vi "2283_catapulta.vi"(1 "swithLimit":bool, 2 "Reset":bool, 3 "catapulta":bool) -> (0 "motor":i32)   [LabVIEW 2015]
uses:
  TypeDefs/estadosCatapulta.ctl
  Globales/Catapulta Disponible Global.vi
panel:
  out "Enum":T1=enum."disparando"
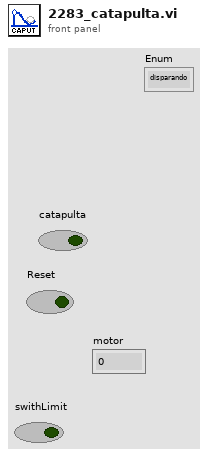
[diagram p1: front panel]
types:
  T1 = typedef "estadosCatapulta.ctl" = enum16{"timeout", "disparando", "cargado"}
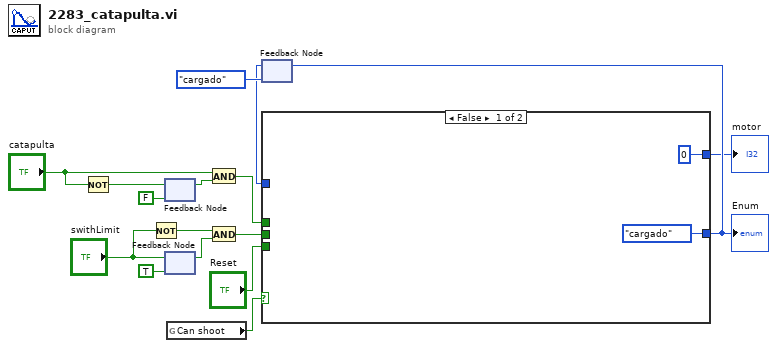
[diagram p0: block diagram]
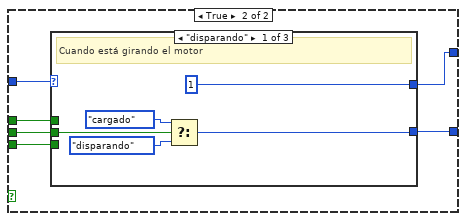
[diagram p2: hidden frame]
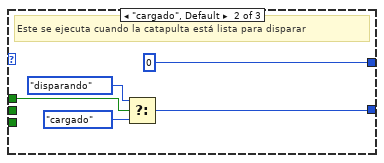
[diagram p3: hidden frame]
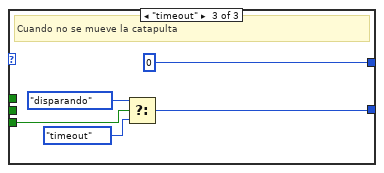
[diagram p4: hidden frame]
diagram:
  n1 = Not(x="catapulta") -> (.not. x?=w11:bool)
  n2 = Not(x="swithLimit") -> (.not. x?=w2:bool)
  n3 = feedback #1(FALSE) -> (w10:bool)
  n4 = feedback-in #1(w11) -> ()
  n5 = feedback #2(TRUE) -> (w7:bool)
  n6 = feedback-in #2("swithLimit") -> ()
  n7 = global read "Catapulta Disponible Global.vi" "Can shoot"() -> (w1:bool)
  n8 = And(x="catapulta", y=w10) -> (x .and. y?=w9:bool)
  n9 = And(x=w2, y=w7) -> (x .and. y?=w6:bool)
  n10 = feedback #3(estadosCatapulta."cargado") -> (w15:T1)
  n11 = case shown="False" w1 {
    tunnel: w15 -> [_ w24]
    tunnel: [estadosCatapulta."cargado" w23] -> w14
    tunnel: [0 w22] -> w13
    tunnel: w9 -> [_ w21]
    tunnel: w6 -> [_ w20]
    tunnel: "Reset" -> [_ w19]
    frame False {
    }
    frame True {
      n12 = case shown="\"disparando\"" w24 {
        tunnel: [w26 w32 w36] -> w23
        tunnel: [1 0 0] -> w22
        tunnel: w21 -> [_ w33 _]
        tunnel: w20 -> [w29 _ _]
        tunnel: w19 -> [_ _ w38]
        frame "disparando" {
          # "Cuando está girando el motor"
          n13 = Select(t=estadosCatapulta."cargado", s=w29, f=estadosCatapulta."disparando") -> (s? t:f=w26:T1)
        }
        frame "cargado", Default {
          # "Este se ejecuta cuando la catapulta está lista para disparar"
          n14 = Select(t=estadosCatapulta."disparando", s=w33, f=estadosCatapulta."cargado") -> (s? t:f=w32:T1)
        }
        frame "timeout" {
          # "Cuando no se mueve la catapulta"
          n15 = Select(t=estadosCatapulta."disparando", s=w38, f=estadosCatapulta."timeout") -> (s? t:f=w36:T1)
        }
      }
    }
  }
  "motor" <- w13
  "Enum" <- w14
  n16 = feedback-in #3(w14) -> ()
